vi "HeaterLoop.vi"(8 "Error In":errorcluster, 10 "Heater Data":refnum<notifier>, 11 "Action Queues":T1) -> (0 "Error Out":errorcluster)   [LabVIEW 2012]
uses:
  ActionQueues.ctl
  UIActionQueueElement.ctl
  UIAction.ctl
  HardwareActionQueueElement.ctl
  HardwareAction.ctl
  HeaterActionQueueElement.ctl
  HeaterAction.ctl
  MFCActionQueueElement.ctl
  MFCAction.ctl
  LogActionQueueElement.ctl
  LogAction.ctl
  <vilib>/Utility/error.llb/DialogType.ctl
  libs/Omega-CSi32/Omega-CSi32.lvlib
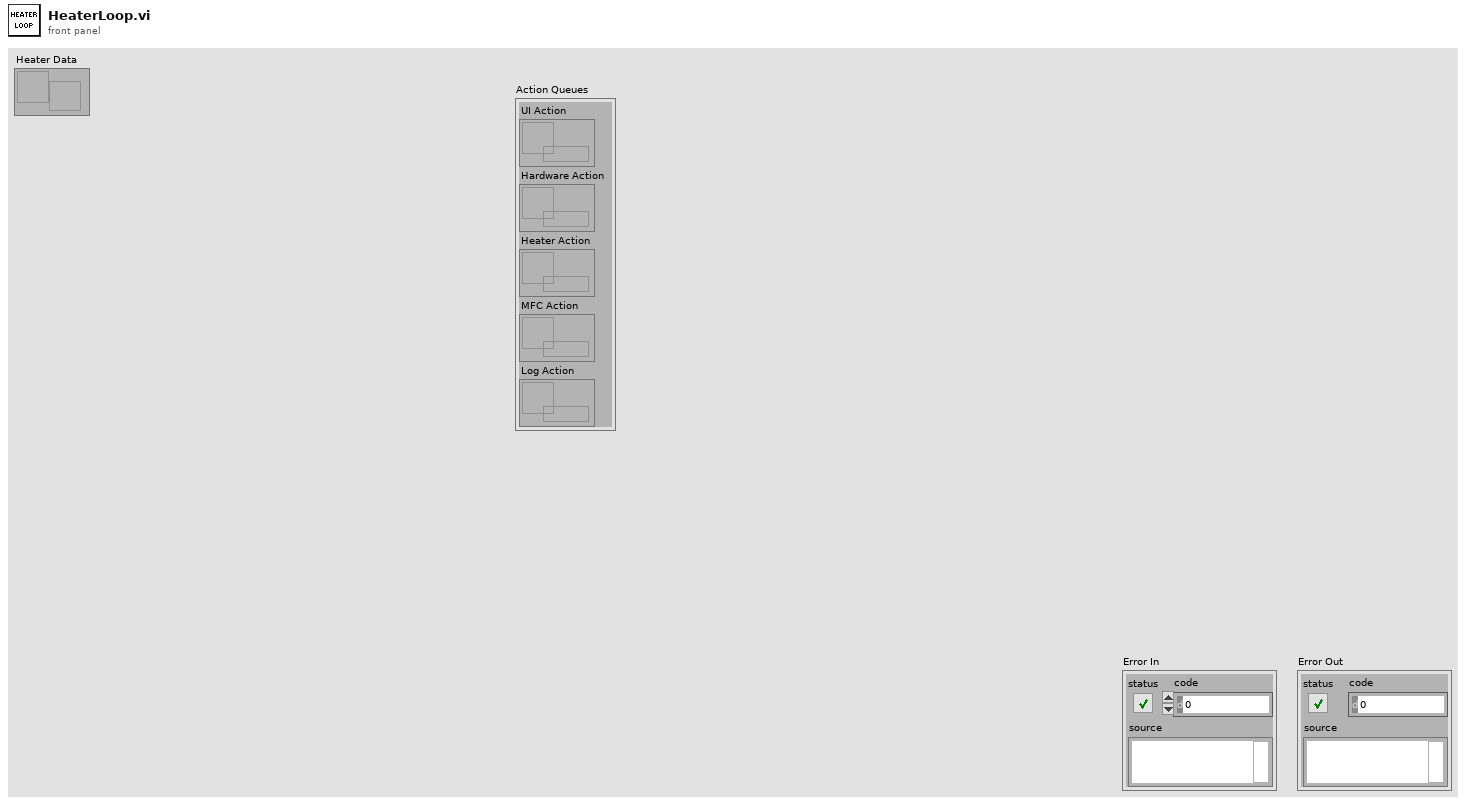
[diagram p1: front panel]
types:
  T1 = typedef "ActionQueues.ctl" = cluster{"UI Action":refnum<queue>, "Hardware Action":refnum<queue>, "Heater Action":refnum<queue>, "MFC Action":refnum<queue>, "Log Action":refnum<queue>}
  T2 = typedef "UIActionQueueElement.ctl" = cluster{"Action":T3, "Data":variant}
  T3 = typedef "UIAction.ctl" = enum16{"Initialize", "Connect", "MFC Connected", "Heater Connected", "Disconnect", "MFC Disconnected", "Heater Disconnected", "Configure MFC", "Configure Heater", "Open Log", "Close Log", "Shutdown"}
  T4 = typedef "HeaterActionQueueElement.ctl" = cluster{"Action":T5, "Data":variant}
  T5 = typedef "HeaterAction.ctl" = enum16{"Initialize", "Start", "Read", "Write", "Stop", "Error", "Shutdown"}
  T6 = typedef "DialogType.ctl" = u16
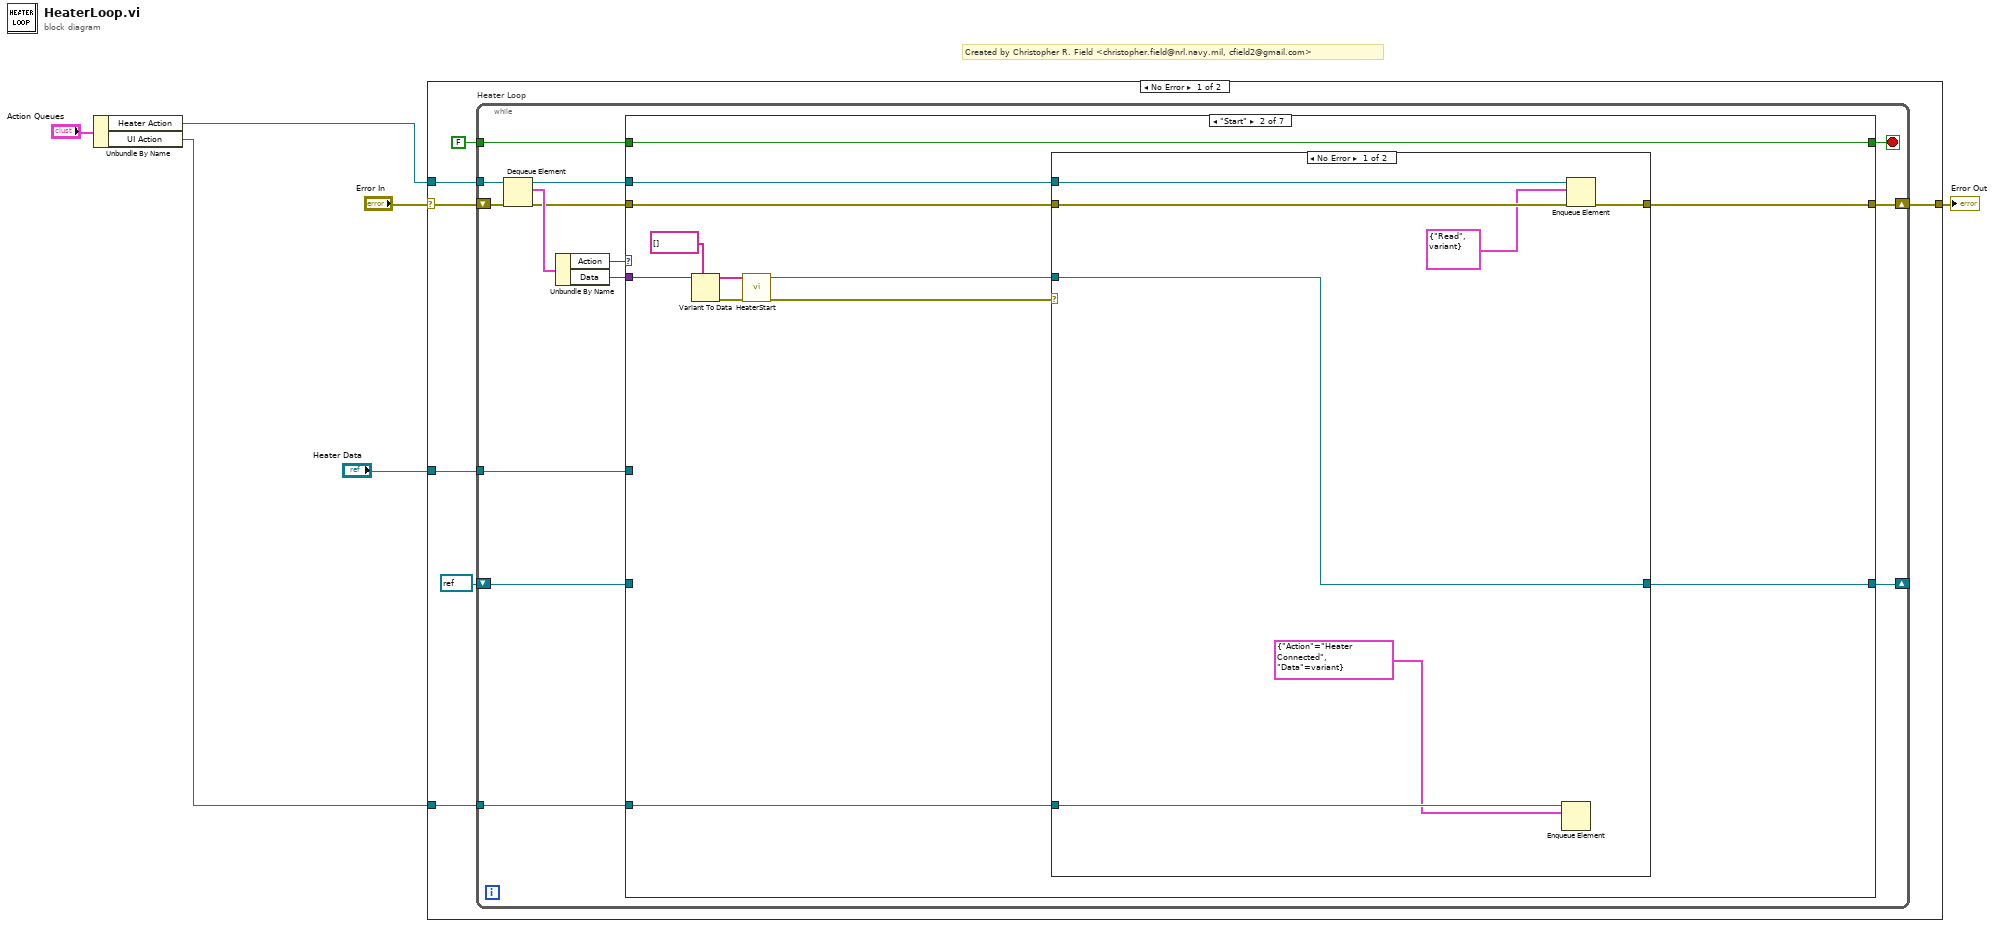
[diagram p0: block diagram]
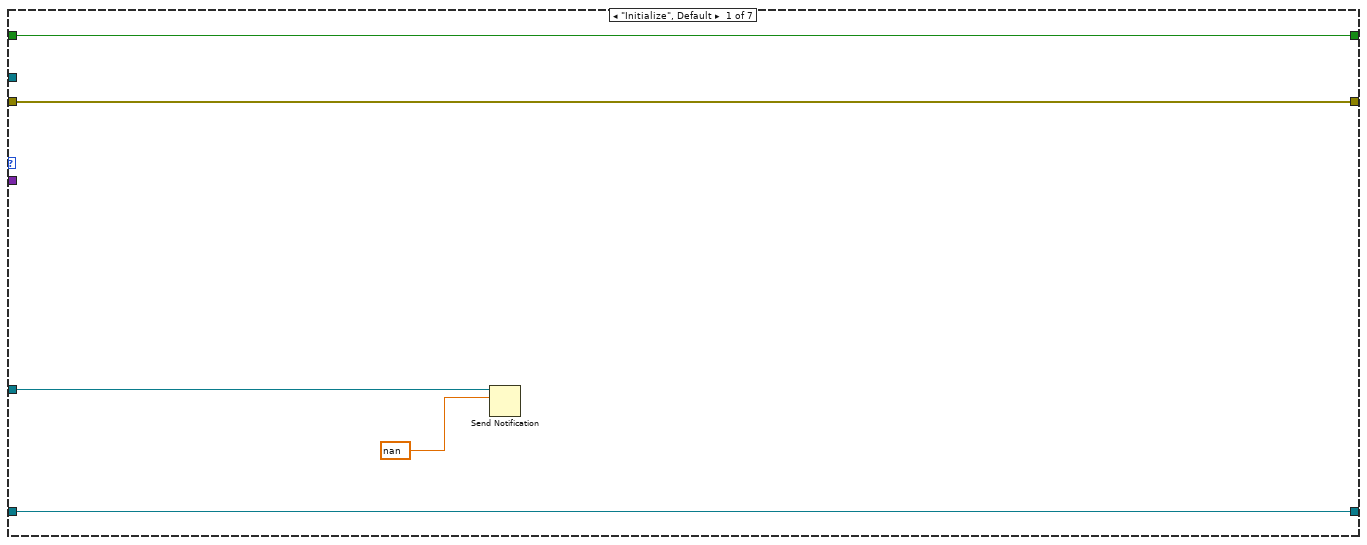
[diagram p2: hidden frame]
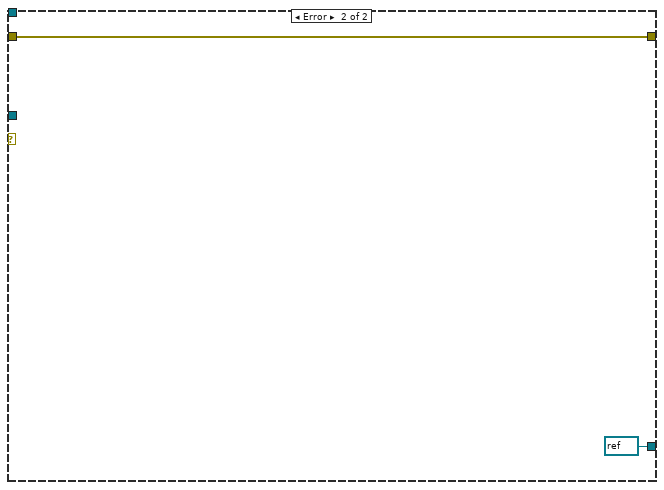
[diagram p3: hidden frame]
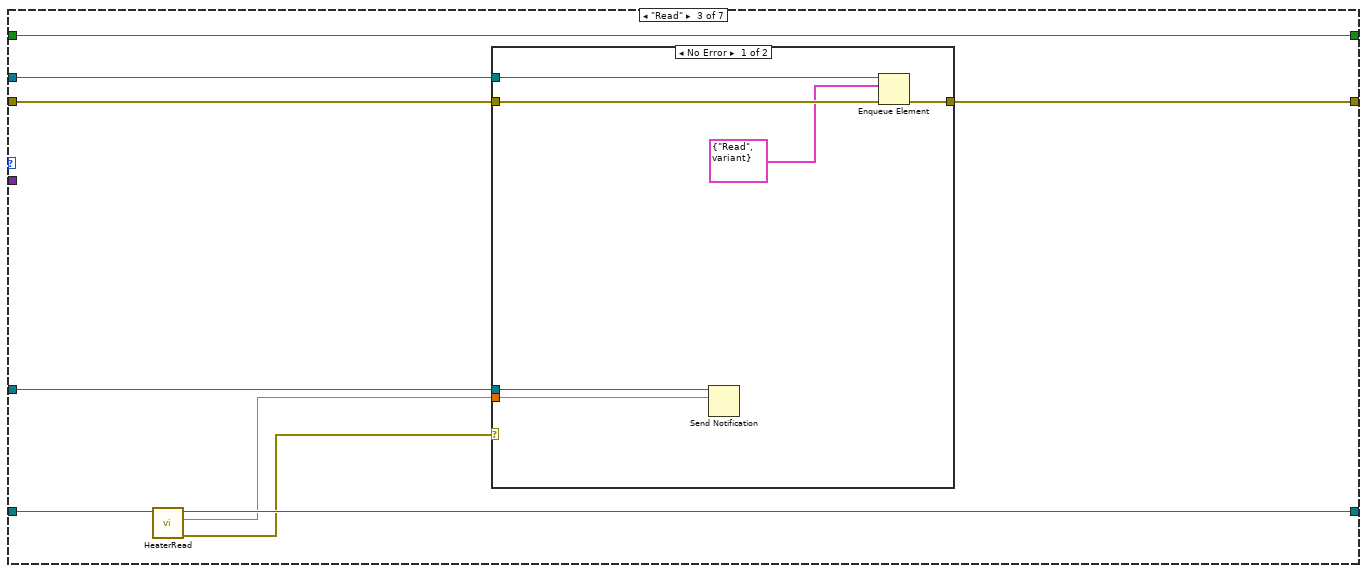
[diagram p4: hidden frame]
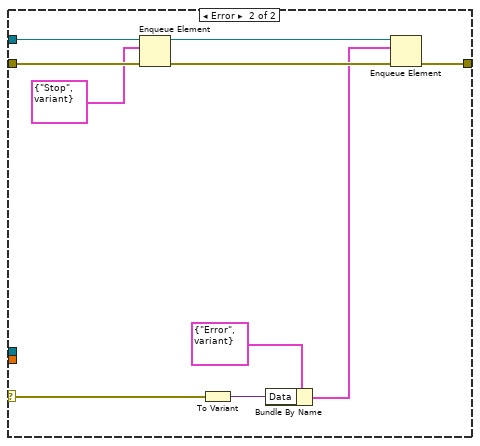
[diagram p5: hidden frame]
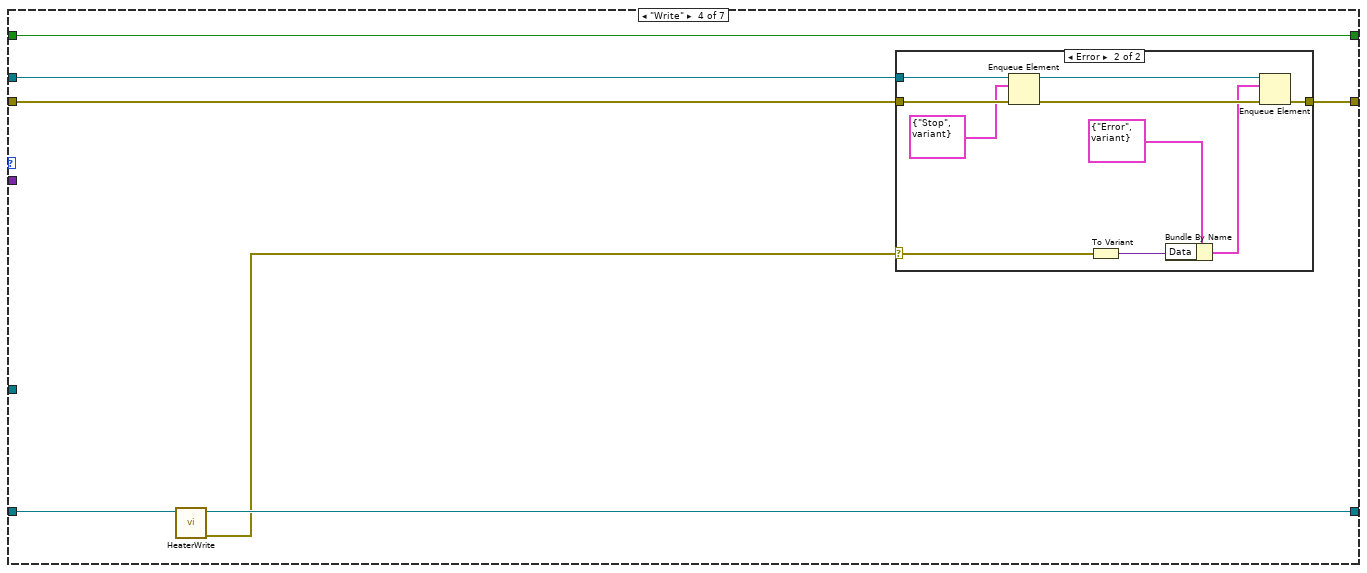
[diagram p6: hidden frame]
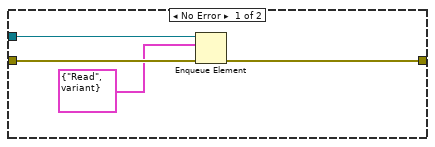
[diagram p7: hidden frame]
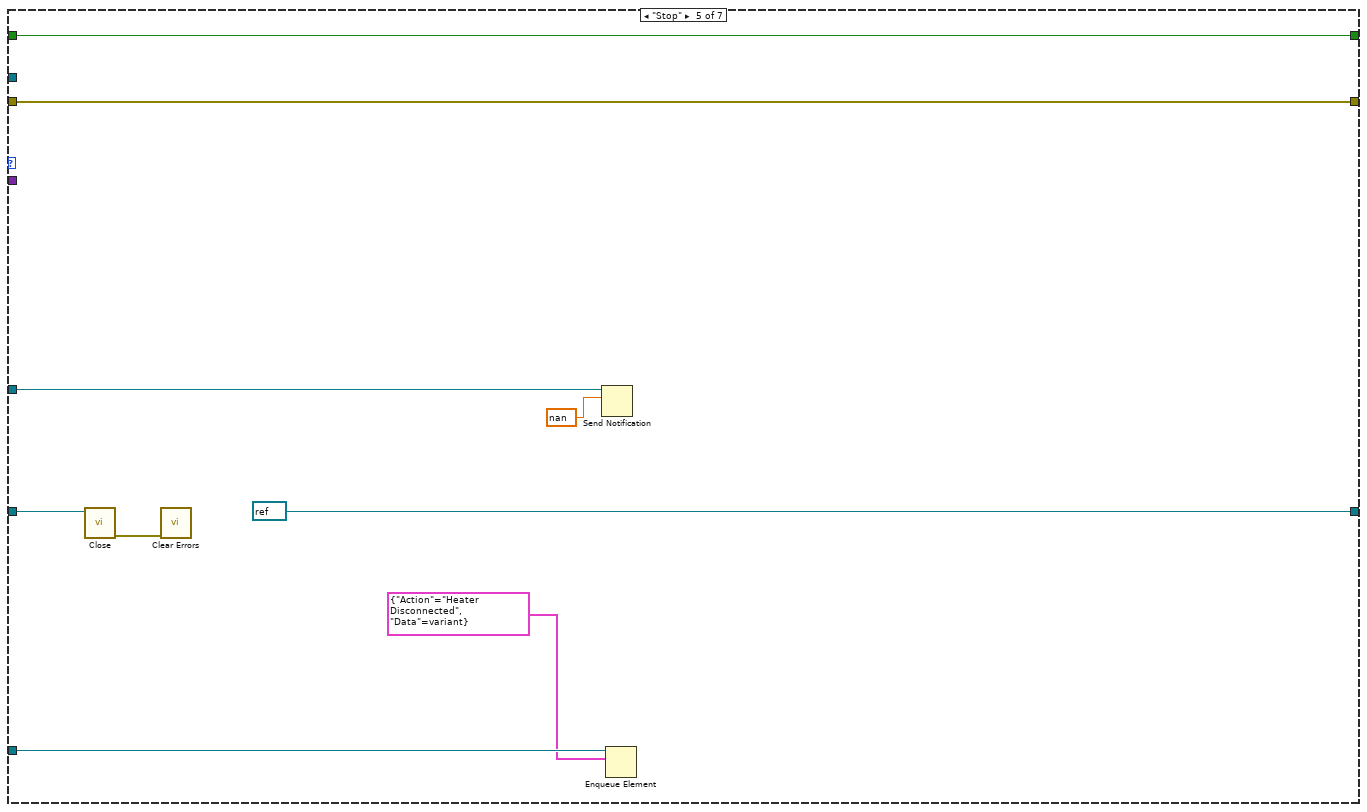
[diagram p8: hidden frame]
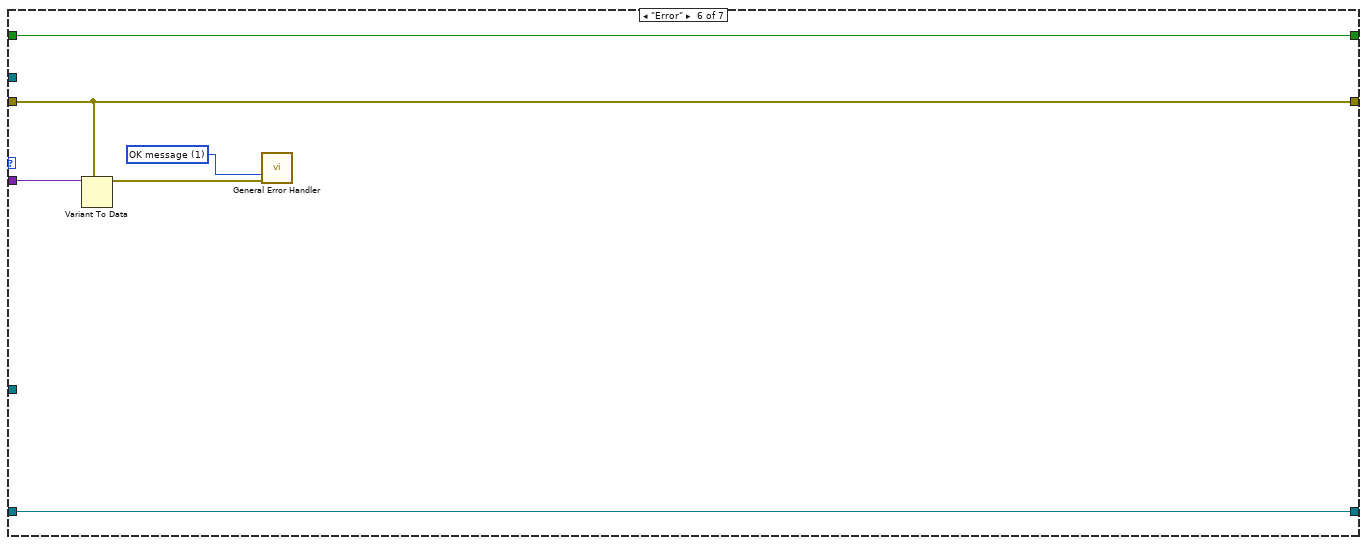
[diagram p9: hidden frame]
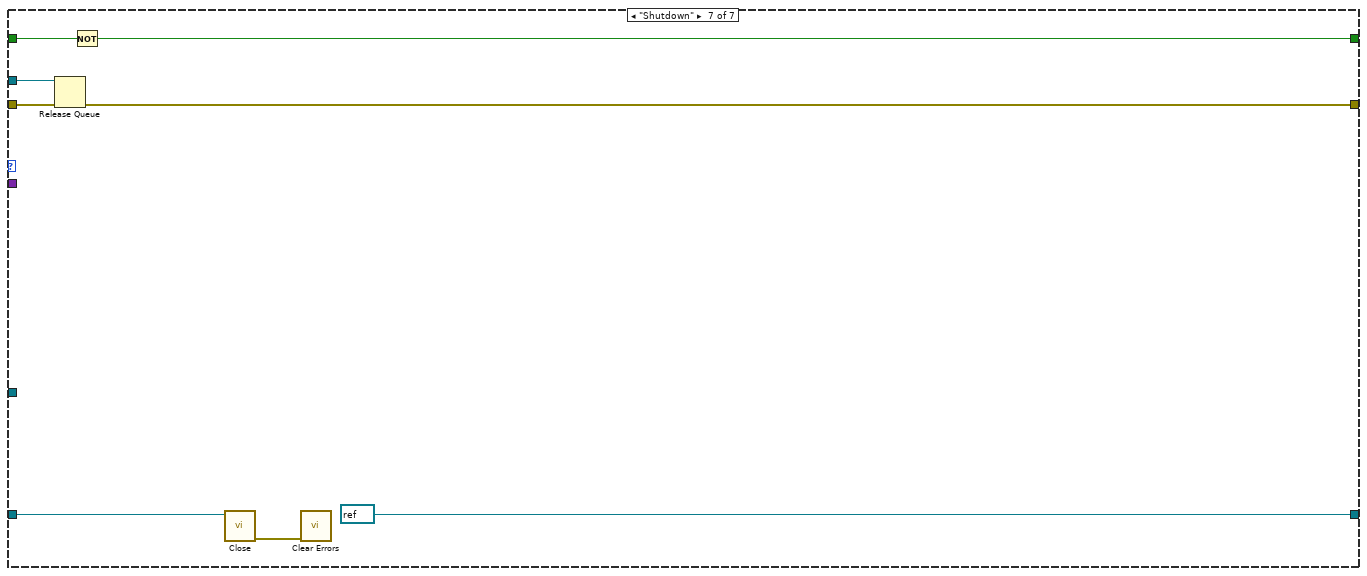
[diagram p10: hidden frame]
diagram:
  # "Created by Christopher R. Field <christopher.field@nrl.navy.mil, cfield2@gmail.com>"
  n1 = Unbundle By Name("Action Queues") -> ("Heater Action"=w3:refnum<queue>, "UI Action"=w2:refnum<queue>)
  n2 = case shown="No Error" "Error In" {
    selector: "Error In" -> [w12 w123]
    tunnel: w3 -> [w11 _]
    tunnel: [w10 w123] -> w5
    tunnel: w2 -> [w8 _]
    tunnel: "Heater Data" -> [w7 _]
    frame No Error {
      n3 = while "Heater Loop" {
        tunnel: FALSE -> [w27]
        shift-right: [w21] -> w10
        shift-left: w12 -> [w26]
        tunnel: w11 -> [w18]
        shift-right: [w17] -> _
        shift-left: refnum<visa-resource-name> refnum ("CSi32 Out") -> [w16]
        tunnel: w8 -> [w15]
        tunnel: w7 -> [w14]
        stop <- w19 stop-if-true
        n4 = Dequeue Element(queue=w18, error in (no error)=w26) -> (queue out=w20:refnum<queue>, element=w25:T4, error out=w22:errorcluster)  [unwired: 1 in, 1 out]
        n5 = Unbundle By Name(w25) -> ("Action"=w24:T5, "Data"=w23:variant)
        n6 = case shown="\"Start\"" w24 {
          tunnel: w27 -> [w31 w44 w62 w85 w108 w114 w122]
          tunnel: w23 -> [_ w38 _ _ _ w112 _]
          tunnel: w22 -> [w32 w41 w60 w83 w107 w111 w119]
          tunnel: [w32 w40 w59 w82 w107 w111 w118] -> w21
          tunnel: w20 -> [_ w42 w61 w84 _ _ w120]
          tunnel: [w31 w44 w62 w85 w108 w114 w121] -> w19
          tunnel: [w30 w43 w57 w80 refnum<visa-resource-name> refnum ("CSi32 Out") w113 refnum<visa-resource-name> refnum ("CSi32 Out")] -> w17
          tunnel: w16 -> [w30 _ w58 w81 w106 w113 w116]
          tunnel: w15 -> [_ w39 _ _ w104 _ _]
          tunnel: w14 -> [w29 _ w54 _ w102 _ _]
          frame "Initialize", Default {
            n7 = Send Notification(notification=nan, notifier=w29) -> ()  [unwired: 1 in, 2 out]
          }
          frame "Start" {
            n8 = Variant To Data(type=string[] [] ("VISA Resource List"), Variant=w38) -> (data=w36:string[], error out=w35:errorcluster)  [unwired: 1 in]
            n9 = call "HeaterStart.vi"("Error In"=w35, "VISA Resource List"=w36) -> ("Error Out"=w34:errorcluster, "Omega CSi32 Out"=w33:refnum<visa-resource-name>)  [unwired: 8 in]
            n10 = case shown="No Error" w34 {
              tunnel: [w45 refnum<visa-resource-name> refnum ("CSi32 Out")] -> w43
              tunnel: w42 -> [w51 _]
              tunnel: w41 -> [w50 w52]
              tunnel: [w49 w52] -> w40
              tunnel: w39 -> [w47 _]
              tunnel: w33 -> [w45 _]
              frame No Error {
                n11 = Enqueue Element(queue=w47, element=T2 {"Action"=enum."Heater Connected", "Data"=variant}) -> ()  [unwired: 2 in, 3 out]
                n12 = Enqueue Element(queue=w51, element=T4 {"Action"=enum."Read", "Data"=variant}, error in (no error)=w50) -> (error out=w49:errorcluster)  [unwired: 1 in, 2 out]
              }
              frame Error {
              }
            }
          }
          frame "Read" {
            n13 = call "HeaterRead.vi"("Omega CSi32 In"=w58) -> ("Error Out"=w56:errorcluster, "Temperature (C)"=w55:dbl, "Omega CSi32 Out"=w57:refnum<visa-resource-name>)  [unwired: 8 in]
            n14 = case shown="No Error" w56 {
              selector: w56 -> [_ w75]
              tunnel: w61 -> [w68 w74]
              tunnel: w60 -> [w67 w73]
              tunnel: [w66 w78] -> w59
              tunnel: w55 -> [w63 _]
              tunnel: w54 -> [w64 _]
              frame No Error {
                n15 = Send Notification(notification=w63, notifier=w64) -> ()  [unwired: 1 in, 2 out]
                n16 = Enqueue Element(queue=w68, element=T4 {"Action"=enum."Read", "Data"=variant}, error in (no error)=w67) -> (error out=w66:errorcluster)  [unwired: 1 in, 2 out]
              }
              frame Error {
                n17 = Enqueue Element(queue=w74, element=T4 {"Action"=enum."Stop", "Data"=variant}, error in (no error)=w73) -> (queue out=w70:refnum<queue>, error out=w71:errorcluster)  [unwired: 1 in, 1 out]
                n18 = To Variant(anything=w75) -> (Variant=w76:variant)
                n19 = Bundle By Name(cluster=T4 {"Action"=enum."Error", "Data"=variant} ("element"), "Data"=w76) -> (w69:T4)
                n20 = Enqueue Element(queue=w70, element=w69, error in (no error)=w71) -> (error out=w78:errorcluster)  [unwired: 1 in, 2 out]
              }
            }
          }
          frame "Write" {
            n21 = call "HeaterWrite.vi"("Omega CSi32 In"=w81) -> ("Error Out"=w79:errorcluster, "Omega CSi32 Out"=w80:refnum<visa-resource-name>)  [unwired: 9 in]
            n22 = case shown="Error" w79 {
              selector: w79 -> [_ w91]
              tunnel: w84 -> [w89 w99]
              tunnel: w83 -> [w88 w98]
              tunnel: [w86 w94] -> w82
              frame No Error {
                n23 = Enqueue Element(queue=w89, element=T4 {"Action"=enum."Read", "Data"=variant}, error in (no error)=w88) -> (error out=w86:errorcluster)  [unwired: 1 in, 2 out]
              }
              frame Error {
                n24 = Enqueue Element(queue=w99, element=T4 {"Action"=enum."Stop", "Data"=variant}, error in (no error)=w98) -> (queue out=w96:refnum<queue>, error out=w95:errorcluster)  [unwired: 1 in, 1 out]
                n25 = To Variant(anything=w91) -> (Variant=w92:variant)
                n26 = Bundle By Name(cluster=T4 {"Action"=enum."Error", "Data"=variant} ("element"), "Data"=w92) -> (w90:T4)
                n27 = Enqueue Element(queue=w96, element=w90, error in (no error)=w95) -> (error out=w94:errorcluster)  [unwired: 1 in, 2 out]
              }
            }
          }
          frame "Stop" {
            n28 = call "Close.vi"("Omega CSi32 In"=w106) -> ("Error Out"=w103:errorcluster)  [unwired: 10 in]
            n29 = call <vilib>:"Clear Errors.vi"("error in (no error)"=w103) -> ()  [unwired: 6 in, 1 out]
            n30 = Send Notification(notification=nan, notifier=w102) -> ()  [unwired: 1 in, 2 out]
            n31 = Enqueue Element(queue=w104, element=T2 {"Action"=enum."Heater Disconnected", "Data"=variant}) -> ()  [unwired: 2 in, 3 out]
          }
          frame "Error" {
            w109 = T6 1 items=["no dialog", "OK message", "continue or stop message", "OK message + warnings", "continue/stop + warnings"] ("type of dialog (OK msg:1)")
            n32 = Variant To Data(type=w111, Variant=w112) -> (data=w110:errorcluster)  [unwired: 1 in, 1 out]
            n33 = call <vilib>:"General Error Handler.vi"("type of dialog (OK msg:1)"=w109, "error in (no error)"=w110) -> ()  [unwired: 9 in, 5 out]
          }
          frame "Shutdown" {
            n34 = Release Queue(queue=w120, error in (no error)=w119) -> (error out=w118:errorcluster)  [unwired: 1 in, 2 out]
            n35 = Not(x=w122) -> (.not. x?=w121:bool)
            n36 = call "Close.vi"("Omega CSi32 In"=w116) -> ("Error Out"=w117:errorcluster)  [unwired: 10 in]
            n37 = call <vilib>:"Clear Errors.vi"("error in (no error)"=w117) -> ()  [unwired: 6 in, 1 out]
          }
        }
      }
    }
    frame Error {
    }
  }
  "Error Out" <- w5
